vi "getEndTone.vi"(8 "error in (no error)":errorcluster, 11 "SingleToneRamp.lvclass in":refnum<class "SingleToneRamp.lvclass">) -> (0 "error out":errorcluster, 2 "endTone":refnum<class "SingleTone.lvclass">, 3 "SingleToneRamp.lvclass out":refnum<class "SingleToneRamp.lvclass">)   [LabVIEW 2009, in "Tools.lvlib" / "Scripting.lvlib" / "SingleToneRamp.lvclass"]
uses:
  SingleToneRamp.lvclass
  SingleTone.lvclass
  SingleToneRamp.lvclass/SingleToneRamp.ctl
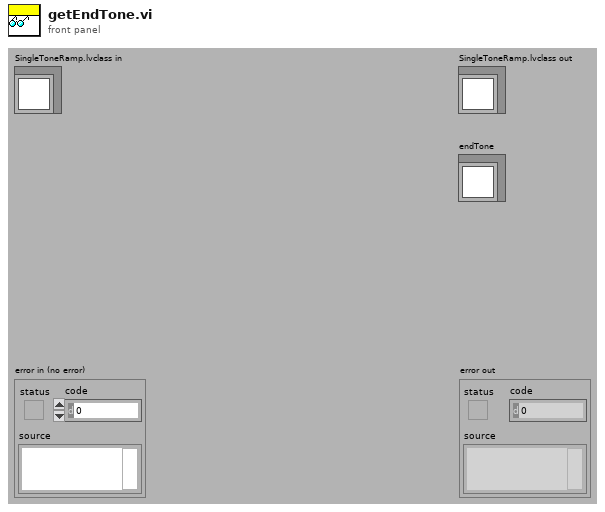
[diagram p1: front panel]
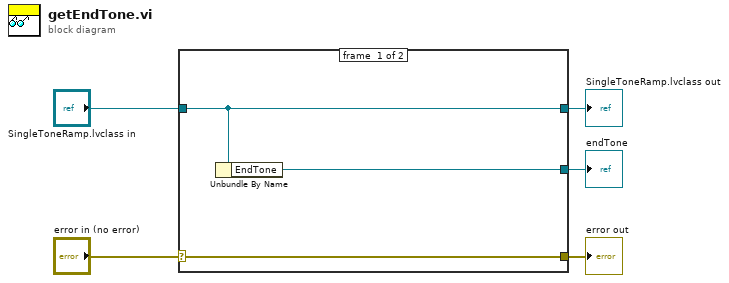
[diagram p0: block diagram]
diagram:
  n1 = case shown="No Error" "error in (no error)" {
    selector: "error in (no error)" -> [w8 w9]
    tunnel: [w8 w9] -> w4
    tunnel: [w7 w10] -> w2
    tunnel: "SingleToneRamp.lvclass in" -> [w7 w10]
    tunnel: [w6 _] -> w1
    frame #0 {
      n2 = Unbundle By Name(w7) -> ("EndTone"=w6:refnum<class "SingleTone.lvclass">)
    }
    frame #1 {
    }
  }
  "error out" <- w4
  "SingleToneRamp.lvclass out" <- w2
  "endTone" <- w1
